vi "gxml_GetTagContents.vi"(7 "Array Container?":bool, 8 "error in":errorcluster, 9 "Item XML":string, 10 "Array Attributes":string, 11 "Item Name/Type":cluster{"Type Enum":T1, "Item Name":string}) -> (0 "error out":errorcluster, 1 "XML After Closing Tag":string, 3 "Item XML Data":T2)   [LabVIEW 2011, in "Third Party VIs.lvlib" / "GXML.lvlib"]
uses:
  GXML.lvlib
  <vilib>/Utility/VariantDataType/Type.ctl
  <vilib>/regexp/Match Regular Expression.xnode
  <vilib>/Utility/VariantDataType/VariantType.lvlib
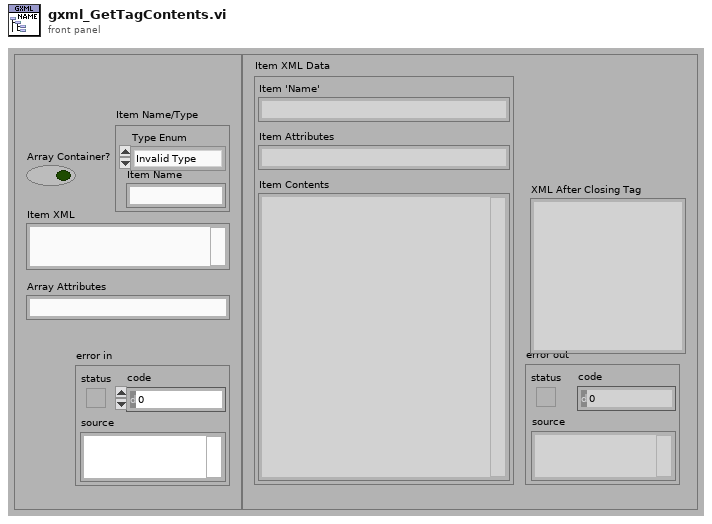
[diagram p1: front panel]
types:
  T1 = typedef "VariantType.lvlib/Type.ctl" = enum8{"Invalid Type", "Void", "I8", "I16", "I32", "I64", "U8", "U16", "U32", "U64", "Single Float", "Double Float", "Extended Float", "Single Complex", "Double Complex", "Extended Complex", "Enum U8", "Enum U16", "Enum U32", "Enum U64", "Single Float With Unit", "Double Float With Unit", "Extended Float With Unit", "Single Complex with Unit", "Double Complex with Unit", "Extended Complex with Unit", "Boolean", "String", "Path", "Picture", "Tag", "Array", "Cluster", "Variant", "LV Variant", "Waveform", "Timestamp", "Digital Waveform", "Digital Data", "ExpressData", "Refnum", "External Data", "VI", "Poly VI", "LabVIEW Class Instance", "Fixed Point"}
  T2 = cluster{"Item 'Name'":string, "Item Attributes":string, "Item Contents":string}
  T3 = cluster{"XML String":string, "XML String":string, "XML String":string}
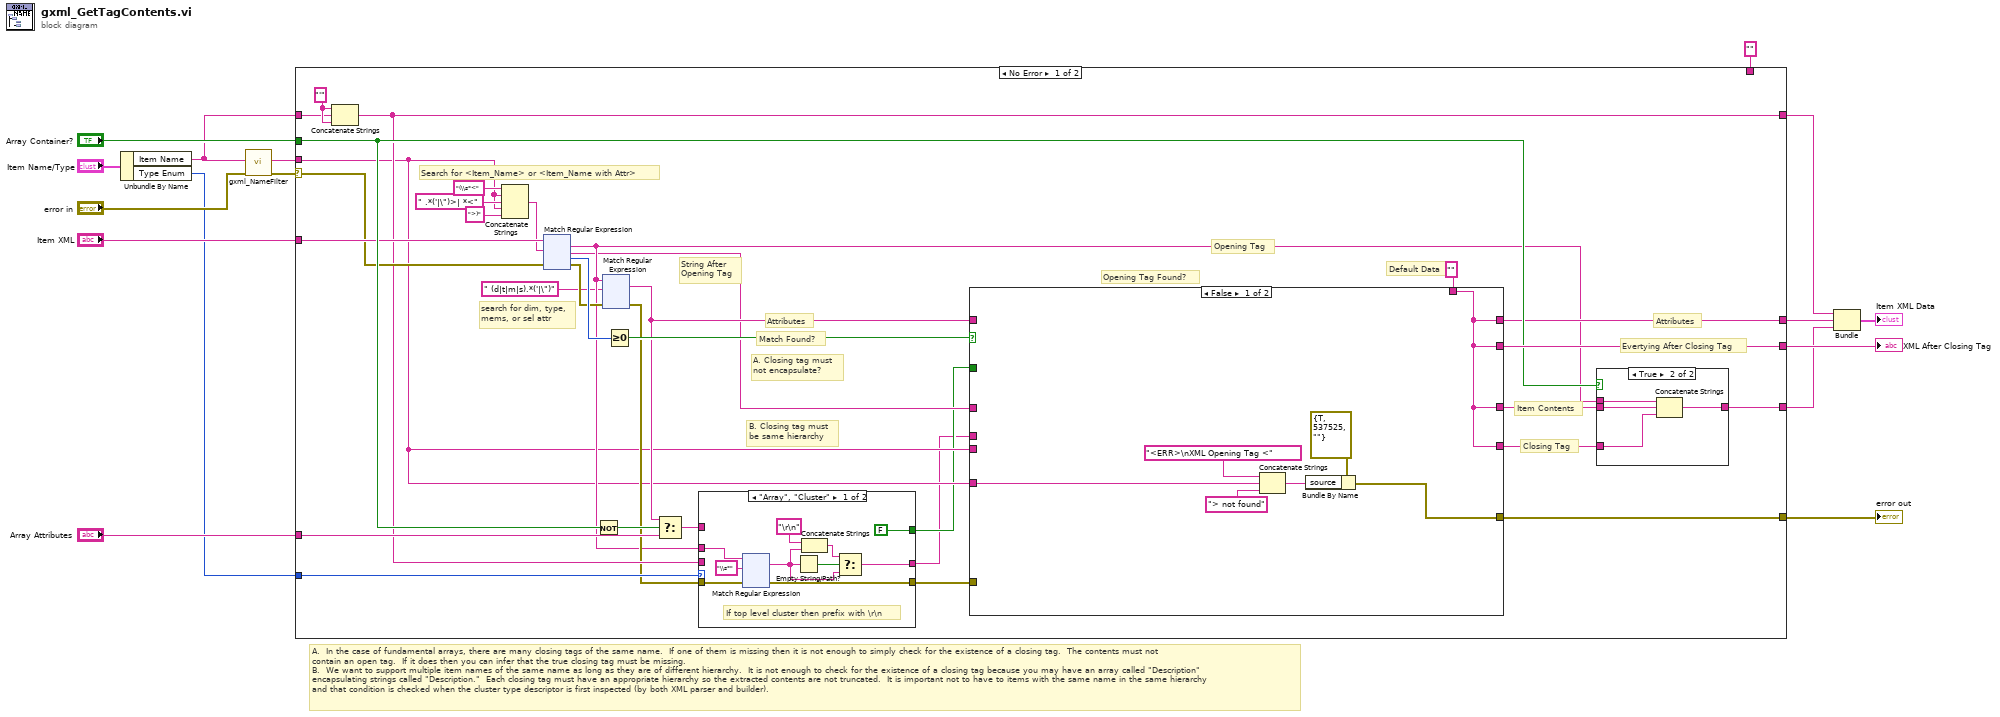
[diagram p0: block diagram]
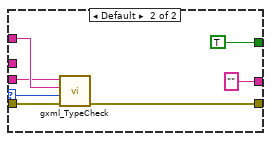
[diagram p2: hidden frame]
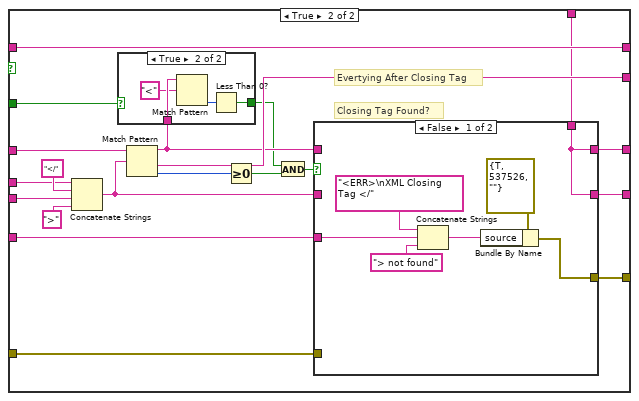
[diagram p4: hidden frame]
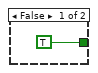
[diagram p5: hidden frame]
diagram:
  # "A.  In the case of fundamental arrays, there are many closing tags of the same name.  If one of them is missing then it is not enough to simply check for the existence of a closing tag.  The contents must not\ncontain an open tag.  If it does then you can infer that the true closing tag must be missing.\nB.  We want to support multiple item names of the same name as long as they are of different hierarchy.  It is not enough to check for the existence of a closing tag because you may have an array called \"Description\"\nencapsulating strings called \"Description.\"  Each closing tag must have an appropriate hierarchy so the extracted contents are not truncated.  It is important not to have to items with the same name in the same hierarchy\nand that condition is checked when the cluster type descriptor is first inspected (by both XML parser and builder)."
  n1 = Unbundle By Name("Item Name/Type") -> ("Item Name"=w4:string, "Type Enum"=w1:T1)
  n2 = call "gxml_NameFilter.vi"("error in"="error in", "Tag Name"=w4) -> ("error out"=w10:errorcluster, "Tag_Name"=w9:string)  [unwired: 7 in]
  n3 = case shown="No Error" w10 {
    selector: w10 -> [w32 w448]
    tunnel: w9 -> [w20 _]
    tunnel: [w48 w447] -> w7
    tunnel: [w42 w447] -> w8
    tunnel: "Item XML" -> [w39 _]
    tunnel: [w28 w448] -> w15
    tunnel: [w49 w447] -> w14
    tunnel: "Array Container?" -> [w43 _]
    tunnel: "Array Attributes" -> [w45 _]
    tunnel: w4 -> [w29 _]
    tunnel: [w26 w447] -> w2
    tunnel: "" ("XML String") -> [_ w447]
    tunnel: w1 -> [w27 _]
    frame No Error {
      w30 = "'" ("string")
      # "A. Closing tag must\nnot encapsulate?"
      # "search for dim, type,\nmems, or sel attr"
      # "Closing Tag"
      # "B. Closing tag must\nbe same hierarchy"
      # "Match Found?"
      # "Attributes"
      # "Search for <Item_Name> or <Item_Name with Attr>"
      # "String After\nOpening Tag"
      # "Evertying After Closing Tag"
      # "Item Contents"
      # "Opening Tag"
      # "Attributes"
      # "Opening Tag Found?"
      # "Default Data"
      n4 = Concatenate Strings(w30, w29, w30) -> (w26:string)
      n5 = Concatenate Strings("(\\s*<", w20, " .*('|\")>| *<" ("regular expression"), w20, ">)" ("regular expression")) -> (w35:string)
      n6 = xnode "Match Regular Expression"("input string"=w39, "regular expression"=w35, "error in"=w32) -> ("whole match"=w23:string, "after match"=w19:string, "offset past match"=w38:i32, "error out"=w33:errorcluster)  [unwired: 3 in, 1 out]
      n7 = Not(x=w43) -> (.not. x?=w44:bool)
      n8 = xnode "Match Regular Expression"("input string"=w23, "regular expression"=" (d|t|m|s).*('|\")", "error in"=w33) -> ("whole match"=w21:string, "error out"=w24:errorcluster)  [unwired: 3 in, 3 out]
      n9 = Greater Or Equal To 0?(x=w38) -> (x >= 0?=w34:bool)
      n10 = Select(t=w21, s=w44, f=w45) -> (s? t:f=w46:string)
      n11 = case shown="\"Array\", \"Cluster\"" w27 {
        selector: w27 -> [_ w395]
        tunnel: w46 -> [_ w399]
        tunnel: [w279 w398] -> w41
        tunnel: w24 -> [w280 w396]
        tunnel: w26 -> [_ w397]
        tunnel: w23 -> [w278 _]
        tunnel: [w275 "" ("whole match")] -> w17
        tunnel: [FALSE TRUE] -> w18
        frame "Array", "Cluster" {
          # "If top level cluster then prefix with \\r\\n"
          n12 = xnode "Match Regular Expression"("input string"=w278, "regular expression"="\\s*", "error in"=w280) -> ("whole match"=w276:string, "error out"=w279:errorcluster)  [unwired: 3 in, 3 out]
          n13 = Empty String/Path?(string/path=w276) -> (empty?=w274:bool)
          n14 = Concatenate Strings("\r\n" ("string"), w276) -> (w272:string)
          n15 = Select(t=w272, s=w274, f=w276) -> (s? t:f=w275:string)
        }
        frame Default {
          n16 = call "gxml_TypeCheck.vi"("error in"=w396, "Type Enum"=w395, "XML Item Attributes"=w399, "Item Name"=w397) -> ("error out"=w398:errorcluster)  [unwired: 7 in]
        }
      }
      n17 = case shown="False" w34 {
        tunnel: [w405 w431] -> w40
        tunnel: w20 -> [w408 w429]
        tunnel: [w407 w430] -> w28
        tunnel: w21 -> [_ w427]
        tunnel: [w405 w427] -> w42
        tunnel: [w405 w426] -> w49
        tunnel: w41 -> [_ w425]
        tunnel: "" ("XML String") -> [w405 w424]
        tunnel: [w405 w423] -> w25
        tunnel: w17 -> [_ w419]
        tunnel: w20 -> [_ w418]
        tunnel: w19 -> [_ w417]
        tunnel: w18 -> [_ w415]
        frame False {
          n18 = Concatenate Strings("<ERR>\nXML Opening Tag <" ("string"), w408, "> not found") -> (w410:string)
          n19 = Bundle By Name(cluster=errorcluster {"status"=TRUE, "code"=537525, "source"=""} ("error IO"), "source"=w410) -> (w407:errorcluster)
        }
        frame True {
          # "Evertying After Closing Tag"
          # "Closing Tag Found?"
          n20 = Concatenate Strings(w419, "</", w418, ">" ("string")) -> (w420:string)
          n21 = Match Pattern(string=w417, regular expression=w420) -> (before substring=w416:string, after substring=w426:string, offset past match=w428:i32)  [unwired: 1 in, 1 out]
          n22 = case shown="True" w415 {
            tunnel: w416 -> [_ w436]
            tunnel: [TRUE w433] -> w413
            frame False {
            }
            frame True {
              n23 = Match Pattern(string=w436, regular expression="<") -> (offset past match=w434:i32)  [unwired: 1 in, 3 out]
              n24 = Less Than 0?(x=w434) -> (x < 0?=w433:bool)
            }
          }
          n25 = Greater Or Equal To 0?(x=w428) -> (x >= 0?=w414:bool)
          n26 = And(x=w413, y=w414) -> (x .and. y?=w412:bool)
          n27 = case shown="False" w412 {
            tunnel: w416 -> [_ w446]
            tunnel: [w437 w446] -> w431
            tunnel: [w440 w445] -> w430
            tunnel: w429 -> [w439 _]
            tunnel: w425 -> [_ w445]
            tunnel: w424 -> [w437 _]
            tunnel: w420 -> [_ w444]
            tunnel: [w437 w444] -> w423
            frame False {
              n28 = Concatenate Strings("<ERR>\nXML Closing Tag </" ("string"), w439, "> not found") -> (w442:string)
              n29 = Bundle By Name(cluster=errorcluster {"status"=TRUE, "code"=537526, "source"=""} ("error IO"), "source"=w442) -> (w440:errorcluster)
            }
            frame True {
              # "Closing Tag"
              # "Item Contents"
            }
          }
        }
      }
      n30 = case shown="True" w43 {
        tunnel: w40 -> [w400 w404]
        tunnel: [w400 w403] -> w48
        tunnel: w23 -> [_ w402]
        tunnel: w25 -> [_ w401]
        frame False {
        }
        frame True {
          n31 = Concatenate Strings(w402, w404, w401) -> (w403:string)
        }
      }
    }
    frame Error {
    }
  }
  "error out" <- w15
  "XML After Closing Tag" <- w14
  n32 = Bundle("XML String"=w2, "XML String"=w8, "XML String"=w7) -> (→"Item XML Data":T3)  [unwired: 1 in]
